vi "FT_Write_Byte_Data.vi"(2 "Bytes To Write":u32, 3 "Buffer":u8[](array[numeric]), 4 "Handle":u32) -> (0 "Bytes Written":u32, 1 "FT_Status":u32)   [LabVIEW 2011]
uses:
  FTD2XX.dll
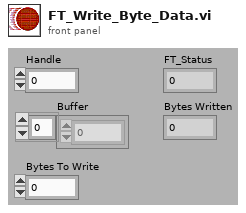
[diagram p1: front panel]
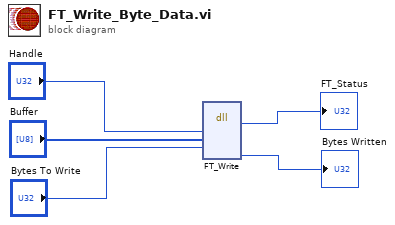
[diagram p0: block diagram]
diagram:
  n1 = dll-call lib="D:/WORK/LabView/#Avesta/D2XX_Functions_7.0/FTD2XX.dll" fn="FT_Write"("Handle"="Handle", "Buffer"="Buffer", "BytesToWrite"="Bytes To Write") -> ("FT_Status"=→"FT_Status":u32, "BytesWritten"=→"Bytes Written":u32)  [unwired: 6 in, 3 out]
